vi "Eliminate duplicate auto-POIs.vi"(9 "Function":T1, 11 "Circles Data in":T2(array[cluster])) -> (2 "empty?":bool, 3 "Circles Data out":T2(array[cluster]))   [LabVIEW 2013]
uses:
  Typedefs/Duplicate POI function enum.ctl
  Global Variables/General Globals.vi
  Program Files (x86)/National Instruments/LabVIEW 2013/user.lib/_OpenG.lib/array/array.llb/Conditional Auto-Indexing Tunnel (Variant)__ogtk.vi
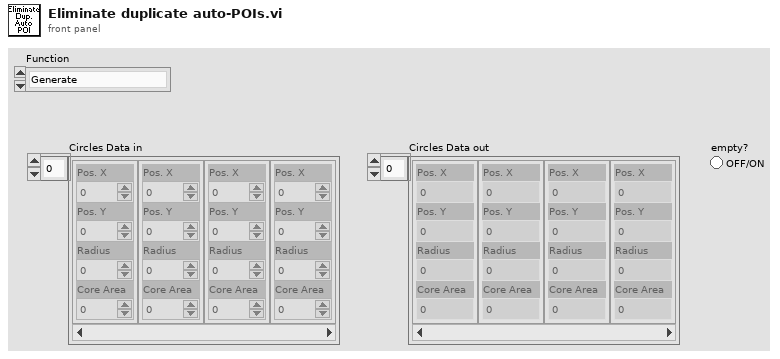
[diagram p1: front panel]
types:
  T1 = typedef "Duplicate POI function enum.ctl" = enum16{"Generate", "Adjust number of POI", "Clear register"}
  T2 = cluster{"Pos. X":i32, "Pos. Y":i32, "Radius":i32, "Core Area":i32}[]
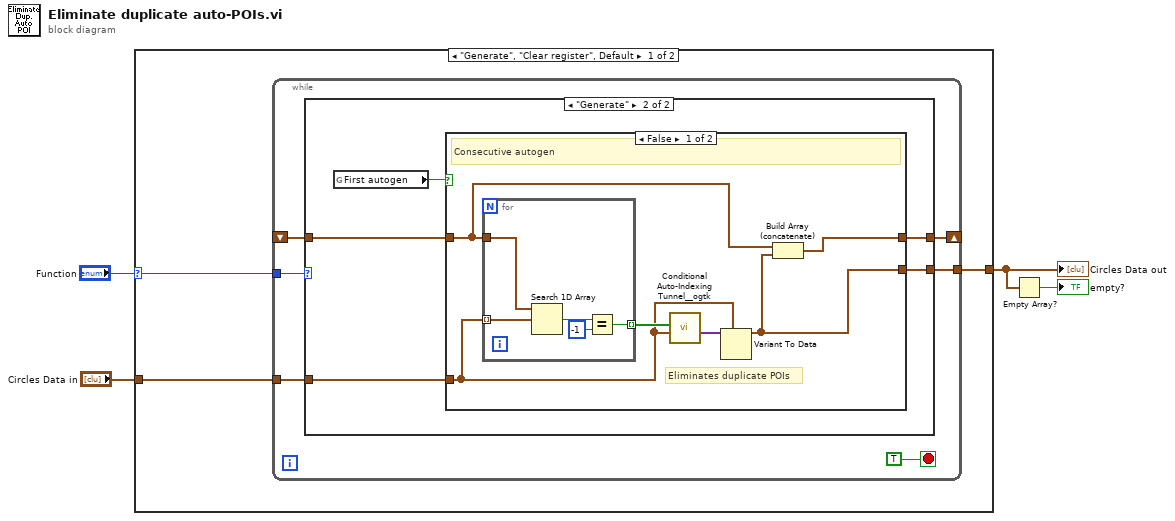
[diagram p0: block diagram]
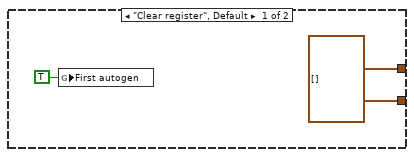
[diagram p2: hidden frame]
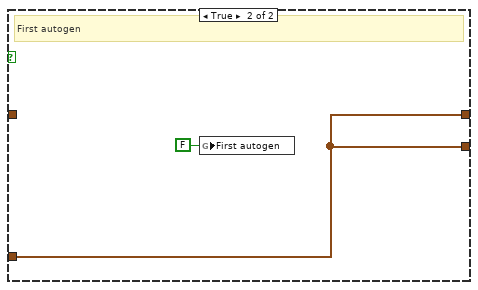
[diagram p3: hidden frame]
diagram:
  n1 = case shown="\"Generate\", \"Clear register\", Default" "Function" {
    selector: "Function" -> [w5 _]
    tunnel: "Circles Data in" -> [w7 w34]
    tunnel: [w6 w34] -> w2
    frame "Generate", "Clear register", Default {
      n2 = while {
        shift-right: [w10] -> _
        shift-left: _ -> [w12]
        tunnel: w7 -> [w9]
        tunnel: [w11] -> w6
        tunnel: w5 -> [w8]
        stop <- TRUE stop-if-true
        n3 = case shown="\"Generate\"" w8 {
          tunnel: w12 -> [_ w20]
          tunnel: [w15 w19] -> w11
          tunnel: [w15 w18] -> w10
          tunnel: w9 -> [_ w17]
          frame "Clear register", Default {
            w15 = T2 [] ("Circles Data in")
            n4 = global write "General Globals.vi" "First autogen"(TRUE ("First autogen")) -> ()
          }
          frame "Generate" {
            n5 = global read "General Globals.vi" "First autogen"() -> (w16:bool)
            n6 = case shown="False" w16 {
              tunnel: [w22 w33] -> w19
              tunnel: w20 -> [w23 _]
              tunnel: [w21 w33] -> w18
              tunnel: w17 -> [w24 w33]
              frame False {
                # "Eliminates duplicate POIs"
                # "Consecutive autogen"
                n7 = for {
                  tunnel: w23 -> [w28]
                  tunnel: [w29] -> w26 mode=indexing
                  tunnel: w24 -> [w27] mode=indexing
                  n8 = Search 1D Array(1D array=w28, element=w27) -> (index of element=w31:i32)  [unwired: 1 in]
                  n9 = Equal?(x=w31, y=-1) -> (x = y?=w29:bool)
                }
                n10 = call-poly "Conditional Auto-Indexing Tunnel__ogtk.vi"("Array in"=w24, "Elements to keep"=w26) -> ("Filtered Array out"=w25:variant[])  [unwired: 5 in]
                n11 = Variant To Data(type=w24, Variant=w25) -> (data=w22:T2)  [unwired: 1 in, 1 out]
                n12 = Build Array (concatenate)(w23, w22) -> (w21:T2)
              }
              frame True {
                # "First autogen"
                n13 = global write "General Globals.vi" "First autogen"(FALSE ("First autogen")) -> ()
              }
            }
          }
        }
      }
    }
    frame "Adjust number of POI" {
    }
  }
  "Circles Data out" <- w2
  n14 = Empty Array?(array=w2) -> (empty?=→"empty?":bool)
